vi "(SubVI) Choose XYZ QPD data.vi"(10 "Filtered QPD data in":dbl[][](array[numeric]), 11 "Axis":enum16{"x", "y", "z"}(ring)) -> (0 "Another Axis Filt. QPD (X or Y)":dbl[](array[numeric]), 3 "Filtered QPD data out":dbl[](array[numeric]))   [LabVIEW 2014]
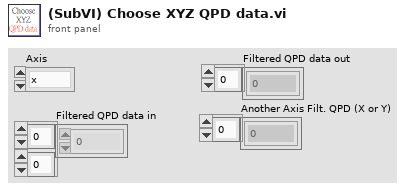
[diagram p1: front panel]
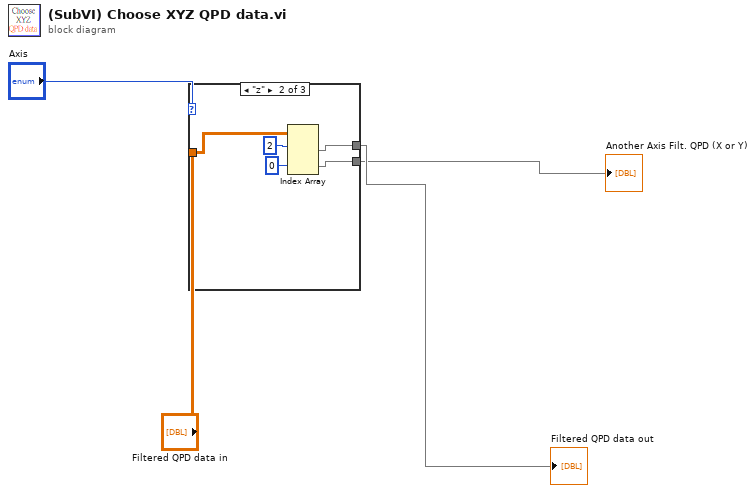
[diagram p0: block diagram]
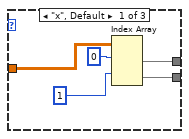
[diagram p2: hidden frame]
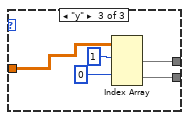
[diagram p3: hidden frame]
diagram:
  n1 = case shown="\"z\"" "Axis" {
    tunnel: [w8 w12 w18] -> w4
    tunnel: "Filtered QPD data in" -> [w7 w13 w17]
    tunnel: [w5 w10 w15] -> w1
    frame "x", Default {
      n2 = Index Array(array=w7, index (row) #1=0 ("index (row)"), index (row) #2=1 ("index (row)")) -> (element #1=w8:dbl[], element #2=w5:dbl[])  [unwired: 2 in]
    }
    frame "z" {
      n3 = Index Array(array=w13, index (row) #1=2 ("index (row)"), index (row) #2=0 ("index (row)")) -> (element #1=w12:dbl[], element #2=w10:dbl[])  [unwired: 2 in]
    }
    frame "y" {
      n4 = Index Array(array=w17, index (row) #1=1 ("index (row)"), index (row) #2=0 ("index (row)")) -> (element #1=w18:dbl[], element #2=w15:dbl[])  [unwired: 2 in]
    }
  }
  "Filtered QPD data out" <- w4
  "Another Axis Filt. QPD (X or Y)" <- w1
